vi "zadanie1.vi"() -> ()   [LabVIEW 2012]
panel:
  out "Wybrana operacja":dbl
  out "Wynik działania:":dbl
  in  "Liczba 2:":dbl
  in  "Liczba 1:":dbl
  in  "Wybierz którą operację chcesz przeprowadzić":u16(ring) items=["działanie 1", "działanie 2", "działanie 3", "działanie 4"]
  # "Program wykonuje jakieś działanie na dwóch liczbach na podstawie elementu wybranego z listy\nSpróbuj zgadnąć jak działa proces wybierania działania"
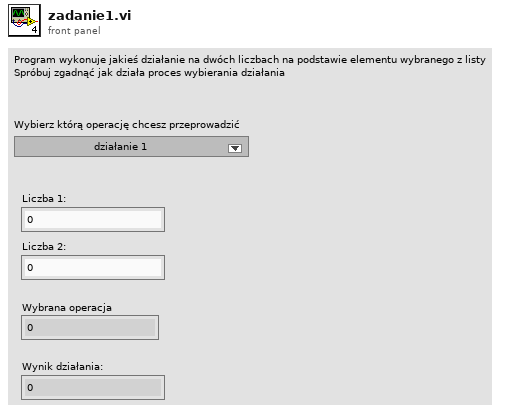
[diagram p1: front panel]
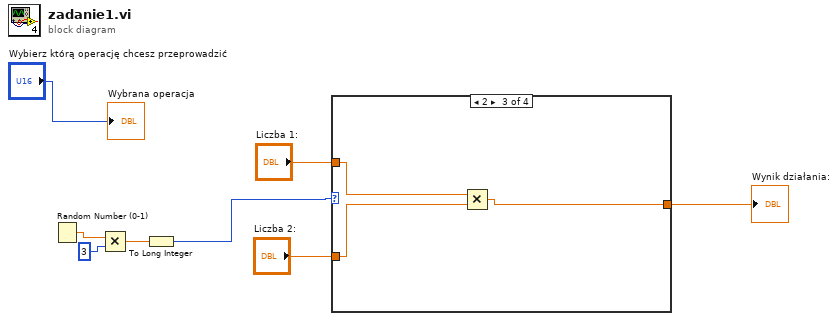
[diagram p0: block diagram]
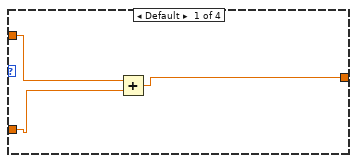
[diagram p2: hidden frame]
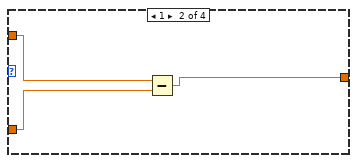
[diagram p3: hidden frame]
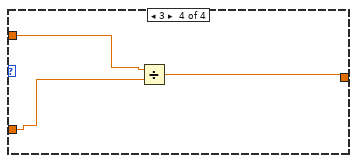
[diagram p4: hidden frame]
diagram:
  n1 = Random Number (0-1)() -> (number: 0 to 1=w5:dbl)
  n2 = Multiply(x=w5, y=3) -> (x*y=w3:dbl)
  n3 = To Long Integer(number=w3) -> (32bit integer=w1:i32)
  n4 = case shown="2" w1 {
    tunnel: "Liczba 2:" -> [w10 w13 w16 w19]
    tunnel: "Liczba 1:" -> [w11 w14 w17 w20]
    tunnel: [w9 w12 w15 w18] -> w6
    frame Default {
      n5 = Add(x=w11, y=w10) -> (x+y=w9:dbl)
    }
    frame 1 {
      n6 = Subtract(x=w14, y=w13) -> (x-y=w12:dbl)
    }
    frame 2 {
      n7 = Multiply(x=w17, y=w16) -> (x*y=w15:dbl)
    }
    frame 3 {
      n8 = Divide(x=w20, y=w19) -> (x/y=w18:dbl)
    }
  }
  "Wynik działania:" <- w6
  "Wybrana operacja" <- "Wybierz którą operację chcesz przeprowadzić"
